vi "RT Loop - Watchdog.vi"(11 "Message Queue":refnum<queue>) -> ()   [LabVIEW 2017]
uses:
  support/Message Queue/Message Cluster.ctl
  <vilib>/RTwatchdog.llb/Watchdog expiration actions.ctl
  <vilib>/RTwatchdog.llb/Watchdog status enum.ctl
  Globals/Global - Configuration Options.vi
  support/Message Queue/Message Queue.lvlib
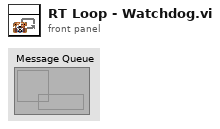
[diagram p1: front panel]
types:
  T1 = typedef "Watchdog status enum.ctl" = enum16{"disabled", "expired", "running"}
  T2 = typedef "Watchdog expiration actions.ctl" = cluster{"reset system":bool, "restart LabVIEW Runtime":bool, "occurrence":bool, "trigger protocol":enum16{"active high", "active low", "open collector"}, "trigger line":enum16{"none", "line 0", "line 1", "line 2", "line 3", "line 4", "line 5", "line 6", "line 7", "SMB line 0"}, "disable watchdog on VI exit":bool}
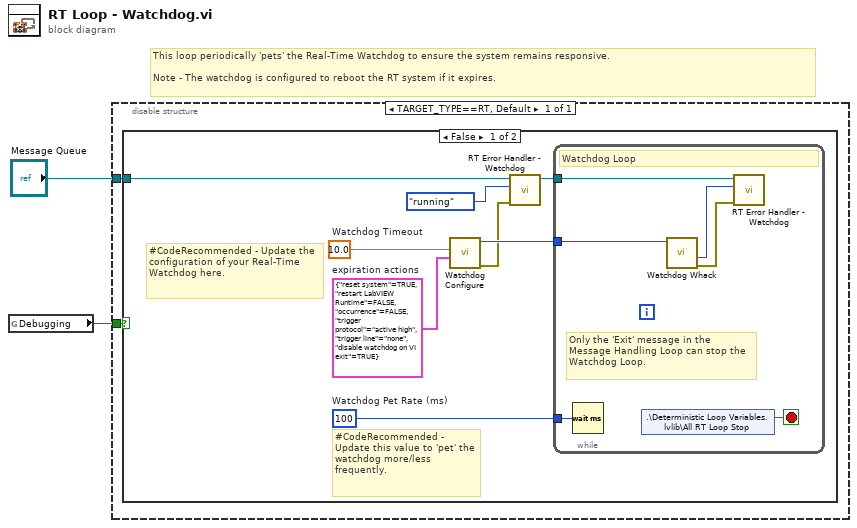
[diagram p0: block diagram]
diagram:
  # "This loop periodically 'pets' the Real-Time Watchdog to ensure the system remains responsive. \n\nNote - The watchdog is configured to reboot the RT system if it expires."
  n1 = global read "Global - Configuration Options.vi" "Debugging"() -> (w1:bool)
  n2 = disable-structure shown="TARGET_TYPE==RT, Default" {
    disable-tunnel: "Message Queue" -> [w4]
    disable-tunnel: w1 -> [w3]
    frame condition #0 (active) {
      n3 = case shown="False" w3 {
        tunnel: w4 -> [w12 _]
        frame False {
          w6 = u32 100  # Watchdog Pet Rate (ms)
          w7 = T2 {"reset system"=TRUE, "restart LabVIEW Runtime"=FALSE, "occurrence"=FALSE, "trigger protocol"=enum."active high", "trigger line"=enum."none", "disable watchdog on VI exit"=TRUE}  # expiration actions
          w8 = 10.0  # Watchdog Timeout
          # "#CodeRecommended - Update the configuration of your Real-Time Watchdog here."
          # "#CodeRecommended - Update this value to 'pet' the watchdog more/less frequently."
          n4 = call <vilib>:"Watchdog Configure.vi"("expiration actions"=w7, "timeout (1 sec)"=w8) -> ("error out"=w9:errorcluster, "watchdogID"=w10:u64)  [unwired: 2 in, 2 out]
          n5 = call "RT Error Handler - Watchdog.vi"("error in (no error)"=w9, "watchdog status"=Watchdog_status_enum."running", "Message Queue"=w12) -> ("dup Message Queue"=w11:refnum<queue>)  [unwired: 8 in]
          n6 = while {
            tunnel: w11 -> [w18]
            tunnel: w10 -> [w16]
            tunnel: w6 -> [w17]
            stop <- w13 stop-if-true
            # "Only the 'Exit' message in the  Message Handling Loop can stop the Watchdog Loop."
            # "Watchdog Loop"
            n7 = Wait (ms)(milliseconds to wait=w17) -> ()  [unwired: 1 out]
            n8 = shared-variable ".\\Deterministic Loop Variables.lvlib\\All RT Loop Stop"() -> (w13:bool)  [unwired: 1 in, 1 out]
            n9 = call <vilib>:"Watchdog Whack.vi"("watchdogID in"=w16) -> ("error out"=w15:errorcluster, "watchdog status"=w14:T1)  [unwired: 4 in, 1 out]
            n10 = call "RT Error Handler - Watchdog.vi"("error in (no error)"=w15, "watchdog status"=w14, "Message Queue"=w18) -> ()  [unwired: 8 in, 1 out]
          }
        }
        frame True {
          # "Do not enable the watchdog when debugging."
        }
      }
    }
  }
